vi "Pressure_Avg.vi"(11 "Pressure_1":sgl[](array[numeric])) -> (3 "Numeric":sgl)   [LabVIEW 2019]
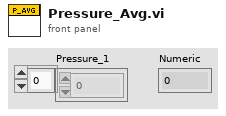
[diagram p1: front panel]
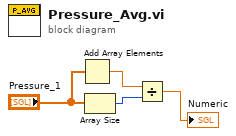
[diagram p0: block diagram]
diagram:
  n1 = Add Array Elements(numeric array="Pressure_1") -> (sum=w3:sgl)
  n2 = Array Size(array="Pressure_1") -> (size(s)=w2:i32)
  n3 = Divide(x=w3, y=w2) -> (x/y=→"Numeric":sgl)
